vi "Prepare Control.vi"(7 "VolatusAPI":refnum<class "VolatusAPI.lvclass">, 8 "error in (no error)":errorcluster, 11 "ValveControl in":refnum<class "InterlockControl.lvclass">) -> (0 "error out":errorcluster, 3 "ValveControl out":refnum<class "InterlockControl.lvclass">)   [LabVIEW 2020, in "VolatusControl.lvlib" / "InterlockControl.lvclass"]
uses:
  InterlockControl.lvclass
  Volatus/VolatusAPI/VolatusAPI.lvclass
  InterlockControl.lvclass/InterlockControl.ctl
  Volatus/VolatusAPI/VolatusAPI.lvclass/VolatusAPI.ctl
  Volatus/Module Identity/Module Identity.lvclass/Module Identity.ctl
  Volatus/Module Identity/Create.vi
  Volatus/Module Identity/Module Identity.lvclass
  C:/dev/lv20CE/relink/lv-volatus/Volatus/Identity/Identity.lvclass
  Volatus/VolatusAPI/Lookup Channel Info.vi
  <vilib>/Utility/error.llb/Error Cluster From Error Code.vi
  Volatus/VolatusAPI/Lookup Q.vi
  lv-vecto/Vecto/ChannelService/Lookup Double Channel.vi
  Volatus/MessageQ/MessageQ.lvclass
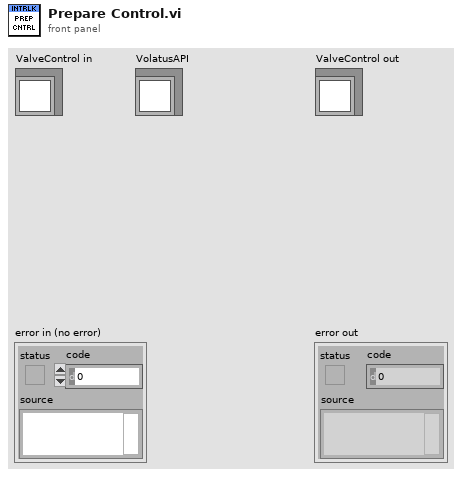
[diagram p1: front panel]
types:
  T1 = typedef "VolatusControl.lvlib/InterlockControl.lvclass/Inhibit Condition.ctl" = cluster{"Channel Name":string, "Comparison":T2, "Value":dbl}
  T2 = typedef "VolatusControl.lvlib/InterlockControl.lvclass/Inhibit Comparison.ctl" = enum16{"Equal", "Less Than", "Greater Than"}
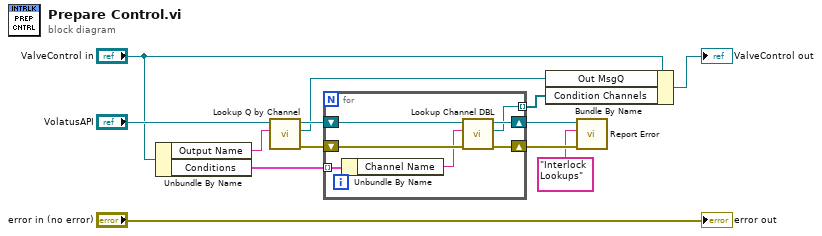
[diagram p0: block diagram]
diagram:
  n1 = Unbundle By Name("ValveControl in") -> ("Output Name"=w9:string, "Conditions"=w6:T1[])
  n2 = call "Lookup Q by Channel.vi"("Channel Name"=w9, "VolatusAPI in"="VolatusAPI") -> ("error out"=w5:errorcluster, "MessageQ"=w7:refnum<class "MessageQ.lvclass">, "VolatusAPI out"=w11:refnum<class "VolatusAPI.lvclass">)  [unwired: 7 in]
  n3 = for {
    tunnel: w6 -> [w18] mode=indexing
    tunnel: [w14] -> w4 mode=indexing
    shift-right: [w16] -> w2
    shift-left: w5 -> [w20]
    shift-right: [w15] -> w3
    shift-left: w11 -> [w19]
    n4 = Unbundle By Name(w18) -> ("Channel Name"=w17:string)
    n5 = call "Lookup Channel DBL.vi"("error in (no error)"=w20, "Name"=w17, "VolatusAPI in"=w19) -> ("error out"=w16:errorcluster, "Channel DBL"=w14:refnum<class "Channel DBL.lvclass">, "VolatusAPI out"=w15:refnum<class "VolatusAPI.lvclass">)  [unwired: 6 in]
  }
  n6 = Bundle By Name(cluster="ValveControl in", "Out MsgQ"=w7, "Condition Channels"=w4) -> (→"ValveControl out":refnum<class "InterlockControl.lvclass">)
  n7 = call "Report Error.vi"("error in (no error)"=w2, "Context"="Interlock Lookups", "VolatusAPI in"=w3) -> ()  [unwired: 7 in, 2 out]
  "error out" <- "error in (no error)"
